vi "USB9825_AD_InitAndRead.vi"(7 "Configuration Parameter":i32[](array[numeric]), 8 "错误输入（无错误）":errorcluster, 9 "READ_MAX_LEN":i32, 10 "DevNum":u8, 11 "hDevice":i32) -> (0 "错误输出":errorcluster, 1 "pBufOver":i32, 2 "通道数":i32, 3 "AD":i16[](array[numeric]))   [LabVIEW 2015, in "DAQ.lvlib"]
uses:
  DAQ.lvlib
  USB9825.DLL
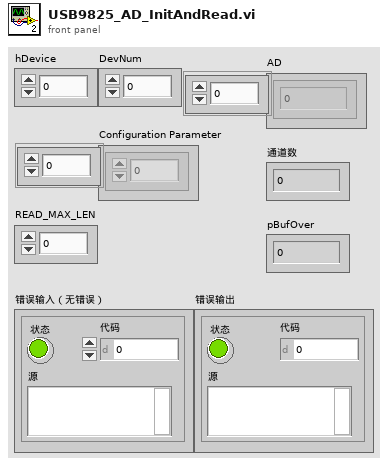
[diagram p1: front panel]
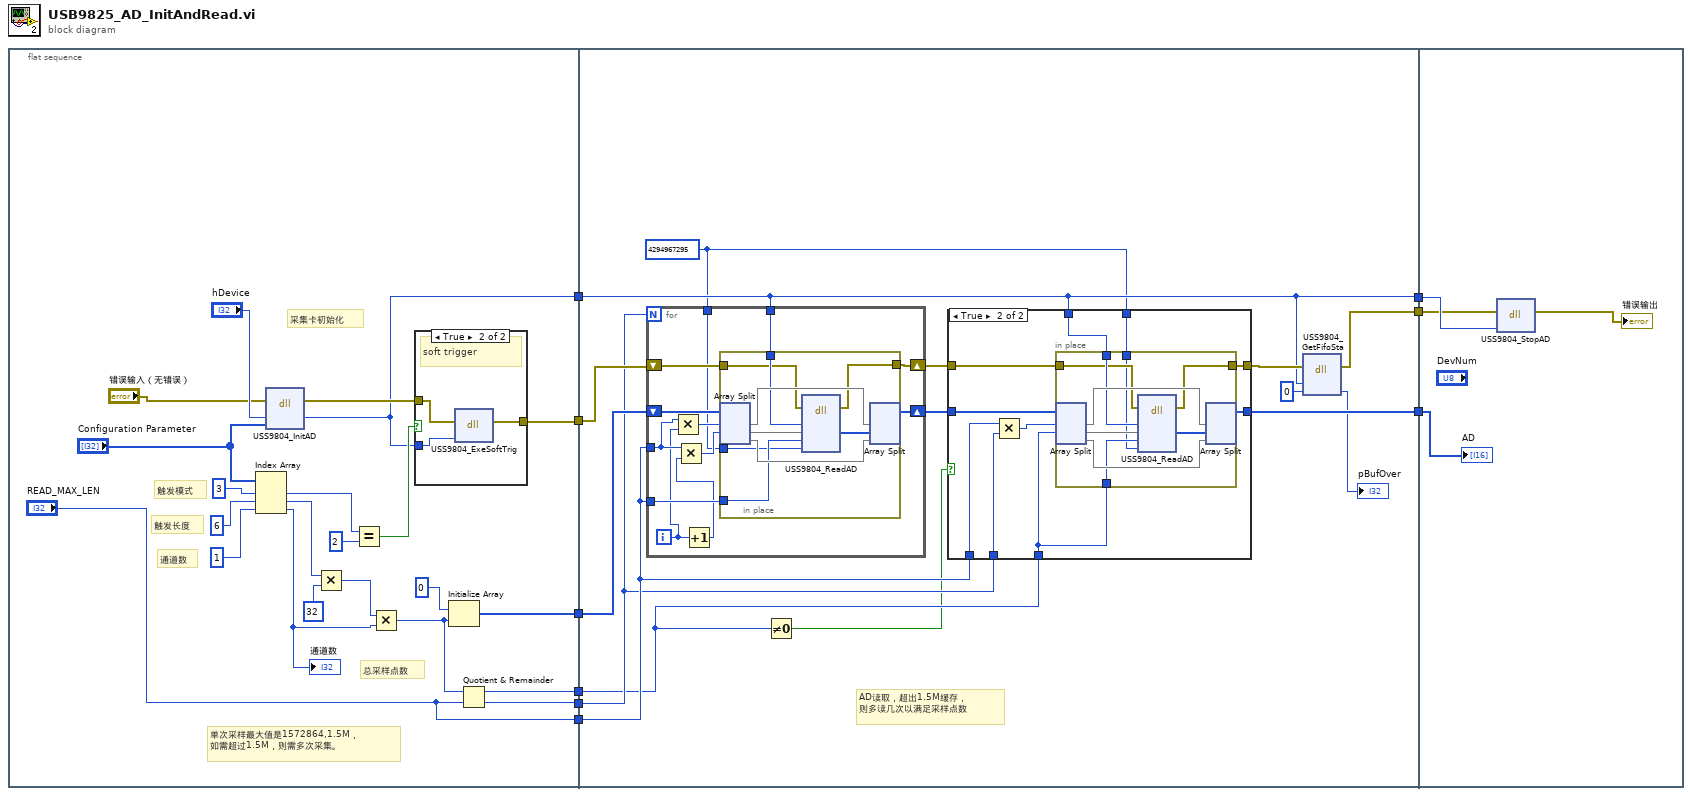
[diagram p0: block diagram]
diagram:
  n1 = flat-sequence {
    tunnel: [w27] -> w9
    tunnel: [w26] -> w8
    tunnel: [w17] -> w6
    tunnel: [w15] -> w5
    tunnel: ["READ_MAX_LEN"] -> w4
    tunnel: [w14] -> w3
    tunnel: w9 -> [w49]
    tunnel: w8 -> [w39]
    tunnel: [w39] -> w7
    tunnel: w6 -> [w50]
    tunnel: w5 -> [w47]
    tunnel: w4 -> [w48]
    tunnel: w3 -> [w46]
    tunnel: [w40] -> w2
    tunnel: [w45] -> w1
    tunnel: w7 -> [w96]
    tunnel: w2 -> [w95]
    tunnel: w1 -> [w94]
    frame #0 {
      # "总采样点数"
      # "通道数"
      # "触发长度"
      # "触发模式"
      # "单次采样最大值是1572864,1.5M，\n如需超过1.5M，则需多次采集。"
      # "采集卡初始化"
      n2 = Index Array(array="Configuration Parameter", index #1=3 ("索引"), index #2=6 ("索引"), index #3=1 ("索引")) -> (element #1=w23:i32, element #2=w21:i32, element #3=w13:i32)
      "通道数" <- w13
      n3 = dll-call lib="PTH2sabs CYexinrongWorkplace\t普密斯Thickness-measurementBiometry_alpha3 bolihouduSub VIsDAQUSB9825.dll" fn="USS9804_InitAD"(error in="错误输入（无错误）", "hDevice"="hDevice", "para_init"="Configuration Parameter") -> (error out=w28:errorcluster, "hDevice"=w26:i32)  [unwired: 4 in, 1 out]
      n4 = Multiply(x=w21, y=32) -> (x*y=w19:i32)
      n5 = Equal?(x=w23, y=u16 2) -> (x = y?=w29:bool)
      n6 = Multiply(x=w19, y=w13) -> (x*y=w16:i32)
      n7 = case shown="True" w29 {
        tunnel: w26 -> [_ w35]
        tunnel: w28 -> [w32 w34]
        tunnel: [w32 w33] -> w27
        frame False {
        }
        frame True {
          # "soft trigger"
          n8 = dll-call lib="PTH2sabs CYexinrongWorkplace\t普密斯Thickness-measurementBiometry_alpha3 bolihouduSub VIsDAQUSB9825.dll" fn="USS9804_ExeSoftTrig"(error in=w34, "hDevice"=w35) -> (error out=w33:errorcluster)  [unwired: 4 in, 1 out]
        }
      }
      n9 = Initialize Array(i16 0 ("元素"), w16) -> (w17:i16[])
      n10 = Quotient & Remainder(x=w16, y="READ_MAX_LEN") -> (x-y*floor(x/y)=w14:i32, floor(x/y)=w15:i32)
    }
    frame #1 {
      w36 = u32 4294967295 ("timeout")
      # "AD读取，超出1.5M缓存，\n则多读几次以满足采样点数"
      n11 = for {
        N: w47 -> [_]
        tunnel: w39 -> [w82]
        tunnel: w48 -> [w80]
        shift-right: [w78] -> w43
        shift-left: w50 -> [w83]
        shift-right: [w79] -> w44
        shift-left: w49 -> [w81]
        tunnel: w48 -> [w75]
        tunnel: w36 -> [w72]
        i -> [w74]
        n12 = Multiply(x=w75, y=w74) -> (x*y=w77:i32)
        n13 = Increment(x=w74) -> (x+1=w73:i32)
        n14 = Multiply(x=w75, y=w73) -> (x*y=w76:i32)
        n15 = in-place {
          in-place-border: w82 -> [w89]
          in-place-border: w81 -> [w88]
          in-place-border: w80 -> [w87]
          in-place-border: [w86] -> w79
          in-place-border: w72 -> [w84]
          n16 = in-place-split #1(w83, w77, w76) -> (w91:i16[], w92:i16[], w90:i16[])
          n17 = dll-call lib="PTH2sabs CYexinrongWorkplace\t普密斯Thickness-measurementBiometry_alpha3 bolihouduSub VIsDAQUSB9825.dll" fn="USS9804_ReadAD"(error in=w88, "hDevice"=w89, "pBuf"=w92, "uCount"=w87, "timeout"=w84) -> (error out=w86:errorcluster, "pBuf"=w85:i16[])  [unwired: 6 in, 1 out]
          n18 = in-place-split #1(w91, w85, w90) -> (w78:i16[])  [unwired: 2 out]
        }
      }
      n19 = Not Equal To 0?(x=w46) -> (x != 0?=w42:bool)
      n20 = case shown="True" w42 {
        tunnel: w44 -> [w52 w62]
        tunnel: w43 -> [w51 w61]
        tunnel: w39 -> [_ w60]
        tunnel: w46 -> [_ w56]
        tunnel: w48 -> [_ w58]
        tunnel: w47 -> [_ w57]
        tunnel: [w52 w55] -> w41
        tunnel: [w51 w54] -> w45
        tunnel: w36 -> [_ w53]
        frame False {
        }
        frame True {
          n21 = Multiply(x=w58, y=w57) -> (x*y=w59:i32)
          n22 = in-place {
            in-place-border: w60 -> [w68]
            in-place-border: w62 -> [w67]
            in-place-border: w56 -> [w66]
            in-place-border: [w64] -> w55
            in-place-border: w53 -> [w63]
            n23 = in-place-split #2(w61, w59, w56) -> (w70:i16[], w71:i16[], w69:i16[])
            n24 = dll-call lib="PTH2sabs CYexinrongWorkplace\t普密斯Thickness-measurementBiometry_alpha3 bolihouduSub VIsDAQUSB9825.dll" fn="USS9804_ReadAD"(error in=w67, "hDevice"=w68, "pBuf"=w71, "uCount"=w66, "timeout"=w63) -> (error out=w64:errorcluster, "pBuf"=w65:i16[])  [unwired: 6 in, 1 out]
            n25 = in-place-split #2(w70, w65, w69) -> (w54:i16[])  [unwired: 2 out]
          }
        }
      }
      n26 = dll-call lib="PTH2sabs CYexinrongWorkplace\t普密斯Thickness-measurementBiometry_alpha3 bolihouduSub VIsDAQUSB9825.dll" fn="USS9804_GetFifoSta"(error in=w41, "hDevice"=w39, "pBufOver"=0) -> (error out=w40:errorcluster, "pBufOver"=→"pBufOver":i32)  [unwired: 4 in, 1 out]
    }
    frame #2 {
      n27 = dll-call lib="PTH2sabs CYexinrongWorkplace\t普密斯Thickness-measurementBiometry_alpha3 bolihouduSub VIsDAQUSB9825.dll" fn="USS9804_StopAD"(error in=w95, "hDevice"=w96) -> (error out=→"错误输出":errorcluster)  [unwired: 4 in, 1 out]
      "AD" <- w94
    }
  }
